vi "TestMatrixMatching.vi"() -> ()   [LabVIEW 2022 SP3]
panel:
  out "Indice":dbl
  out "# thermistance":dbl
  in  "stop":bool
  out "Intensity Graph":dbl[][](graph)
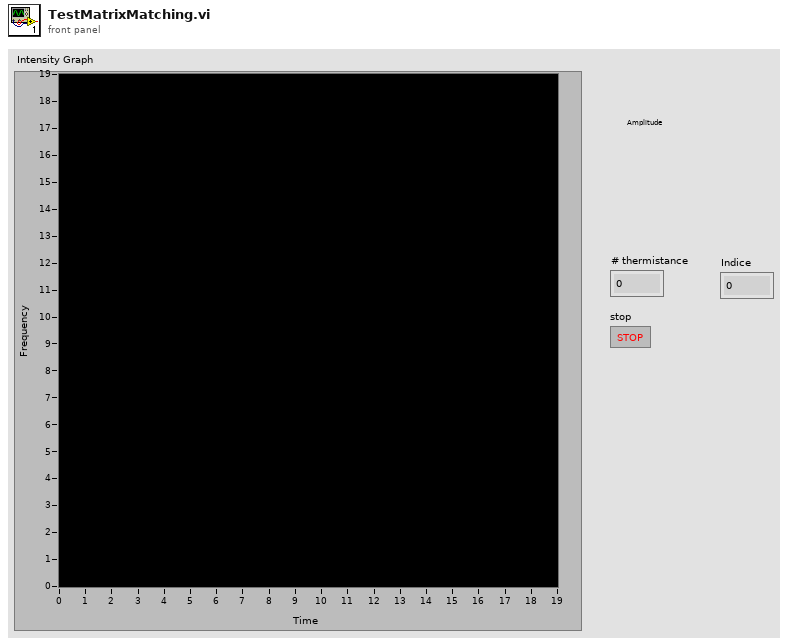
[diagram p1: front panel]
types:
  T1 = enum16{"open", "replace", "create", "open or create", "replace or create", "replace or create with confirmation"}
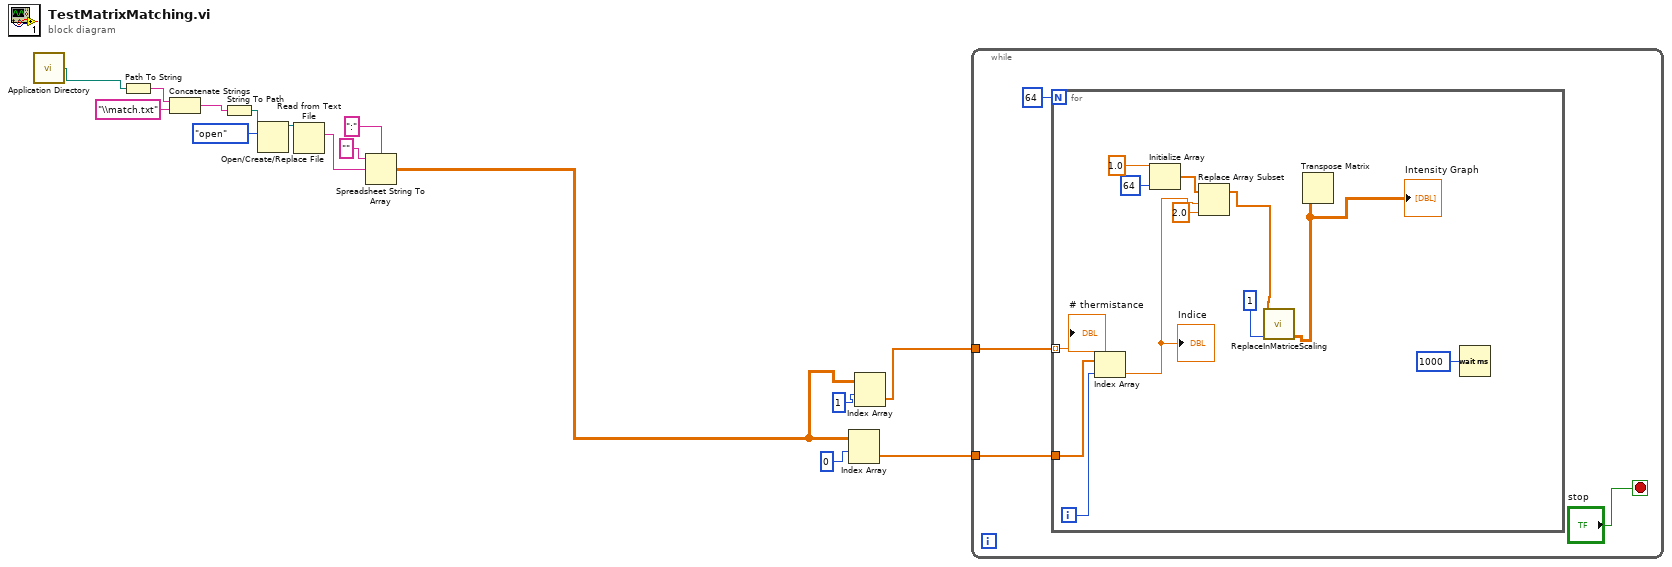
[diagram p0: block diagram]
diagram:
  n1 = call <vilib>:"Application Directory.vi"() -> ("Application Directory"=w7:path)
  n2 = Path To String(path=w7) -> (string=w15:string)
  n3 = Concatenate Strings(w15, "\\match.txt" ("string")) -> (w13:string)
  n4 = String To Path(string=w13) -> (path=w12:path)
  n5 = Open/Create/Replace File(file path (use dialog)=w12, operation (0:open)=T1."open") -> (refnum out=w10:refnum<file>)  [unwired: 4 in, 2 out]
  n6 = Read from Text File(file (use dialog)=w10) -> (text=w9:string)  [unwired: 3 in, 3 out]
  n7 = Spreadsheet String To Array(delimiter (Tab)=":", format string="", spreadsheet string=w9) -> (array=w6:dbl[][])  [unwired: 1 in]
  n8 = Index Array(array=w6, index (row)=0 ("disabled index (col)")) -> (element=w5:dbl[])  [unwired: 1 in]
  n9 = Index Array(array=w6, index (row)=1 ("index (col)")) -> (element=w4:dbl[])  [unwired: 1 in]
  n10 = while {
    tunnel: w5 -> [w17]
    tunnel: w4 -> [w16]
    stop <- "stop" stop-if-true
    n11 = for {
      N: 64 -> [_]
      tunnel: w17 -> [w24]
      tunnel: w16 -> [w21] mode=indexing
      i -> [w23]
      n12 = Index Array(array=w24, index=w23) -> (element=w22:dbl)
      "Indice" <- w22
      n13 = Initialize Array(1.0 ("element"), 64 ("dimension size")) -> (w27:dbl[])
      n14 = Replace Array Subset(array=w27, new element=2.0 ("new element/subarray"), index=w22) -> (w25:dbl[])
      n15 = call "ReplaceInMatriceScaling.vi"("Input Scaling"=1, "Input Array"=w25) -> ("Output Array"=w29:dbl[][])  [unwired: 9 in]
      "Intensity Graph" <- w29
      n16 = Transpose Matrix(1:w29) -> ()  [unwired: 1 out]
      n17 = Wait (ms)(milliseconds to wait=u32 1000) -> ()  [unwired: 1 out]
      "# thermistance" <- w21
    }
  }
